vi "Diagram Get Constant Assignements.vi"(11 "Diagram ref.":refnum<vi>) -> (3 "Constant assignements to wires":string)   [LabVIEW 2014]
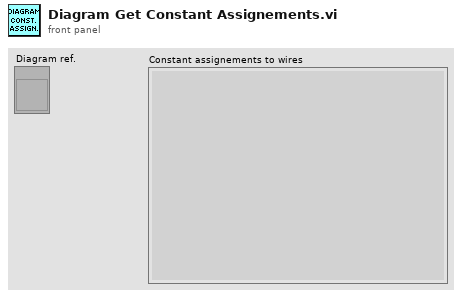
[diagram p1: front panel]
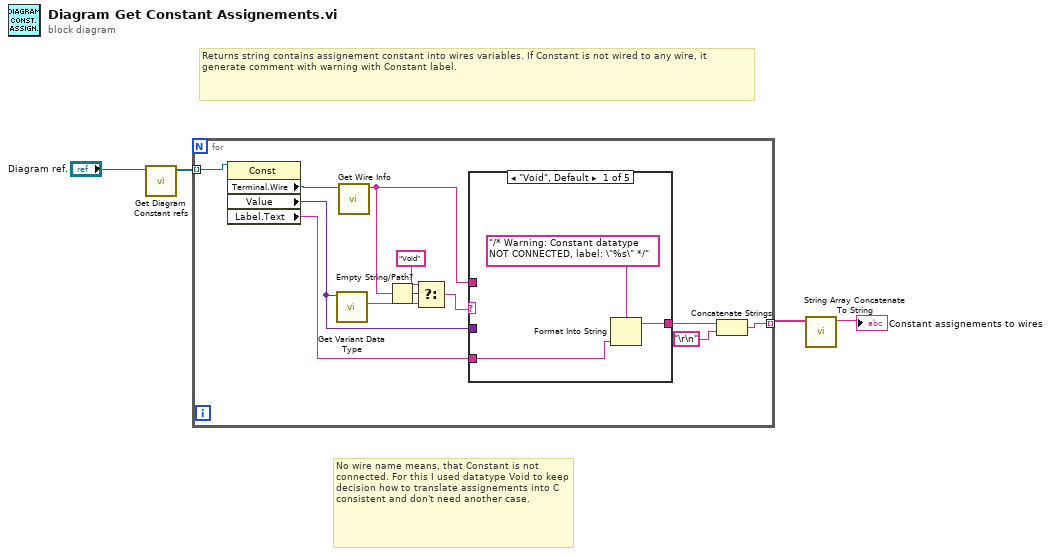
[diagram p0: block diagram]
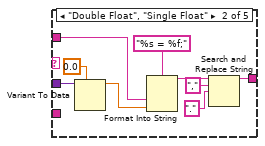
[diagram p2: hidden frame]
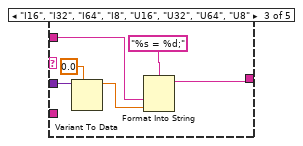
[diagram p3: hidden frame]
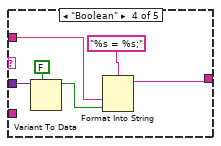
[diagram p4: hidden frame]
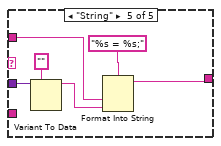
[diagram p5: hidden frame]
diagram:
  # "No wire name means, that Constant is not connected. For this I used datatype Void to keep decision how to translate assignements into C consistent and don't need another case."
  # "Returns string contains assignement constant into wires variables. If Constant is not wired to any wire, it generate comment with warning with Constant label."
  n1 = call "Get Diagram Constant refs.vi"("Diagram ref."="Diagram ref.") -> ("Constant"=w3:refnum<vi>[])  [unwired: 10 in]
  n2 = for {
    tunnel: [w15] -> w2 mode=indexing
    tunnel: w3 -> [w13] mode=indexing
    n3 = property class="Const"(reference=w13) -> ("Terminal.Wire"=w16:refnum<vi>, "Value"=w11:variant, "Label.Text"=w5:string)  [unwired: 1 in, 2 out]
    n4 = call "Get Variant Data Type.vi"("Variant in"=w11) -> ("first data type"=w9:string)  [unwired: 9 in, 1 out]
    n5 = call "Get Wire Info.vi"("Wire"=w16) -> ("wire label"=w7:string)  [unwired: 9 in, 1 out]
    n6 = Empty String/Path?(string/path=w7) -> (empty?=w10:bool)
    n7 = Select(t="Void", s=w10, f=w9) -> (s? t:f=w6:string)
    n8 = case shown="\"Void\", Default" w6 {
      tunnel: w11 -> [_ w23 w31 w38 w45]
      tunnel: w7 -> [_ w21 w29 w36 w43]
      tunnel: [w18 w20 w34 w40 w41] -> w12
      tunnel: w5 -> [w17 _ _ _ _]
      frame "Void", Default {
        n9 = Format Into String(format string="/* Warning: Constant datatype NOT CONNECTED, label: \"%s\" */" ("result string"), w17) -> (resulting string=w18:string)  [unwired: 2 in, 1 out]
      }
      frame "Double Float", "Single Float" {
        n10 = Variant To Data(type=0.0, Variant=w23) -> (data=w22:dbl)  [unwired: 1 in, 1 out]
        n11 = Format Into String(format string="%s = %f;", w21, w22) -> (resulting string=w26:string)  [unwired: 2 in, 1 out]
        n12 = Search and Replace String(input string=w26, search string=",", replace string="." ("search string")) -> (result string=w20:string)  [unwired: 5 in, 3 out]
      }
      frame "I16", "I32", "I64", "I8", "U16", "U32", "U64", "U8" {
        n13 = Variant To Data(type=0.0, Variant=w31) -> (data=w30:dbl)  [unwired: 1 in, 1 out]
        n14 = Format Into String(format string="%s = %d;", w29, w30) -> (resulting string=w34:string)  [unwired: 2 in, 1 out]
      }
      frame "Boolean" {
        n15 = Variant To Data(type=FALSE, Variant=w38) -> (data=w37:bool)  [unwired: 1 in, 1 out]
        n16 = Format Into String(format string="%s = %s;", w36, w37) -> (resulting string=w40:string)  [unwired: 2 in, 1 out]
      }
      frame "String" {
        n17 = Variant To Data(type="", Variant=w45) -> (data=w44:string)  [unwired: 1 in, 1 out]
        n18 = Format Into String(format string="%s = %s;", w43, w44) -> (resulting string=w41:string)  [unwired: 2 in, 1 out]
      }
    }
    n19 = Concatenate Strings(w12, "\r\n") -> (w15:string)
  }
  n20 = call "String Array Concatenate To String.vi"("Array String In"=w2) -> ("String"=→"Constant assignements to wires":string)  [unwired: 10 in]
